vi "Mass Assign Window Text.vi"() -> ()   [LabVIEW 2023]
uses:
  9ee1baf5-252d-4dbe-adf5-4428d1966d26.vi
  96e9d38a-46f1-45bd-90ed-3046ef3e3c05.vi
  <userlib>/_OpenG.lib/file/file.llb/openg_file.lvlib
panel:
  out "file paths":path[](array[path])
  out "error out":errorcluster
  out "N":i32
  out "i":i32
  in  "error in (no error)":errorcluster
  in  "Decal Root":path
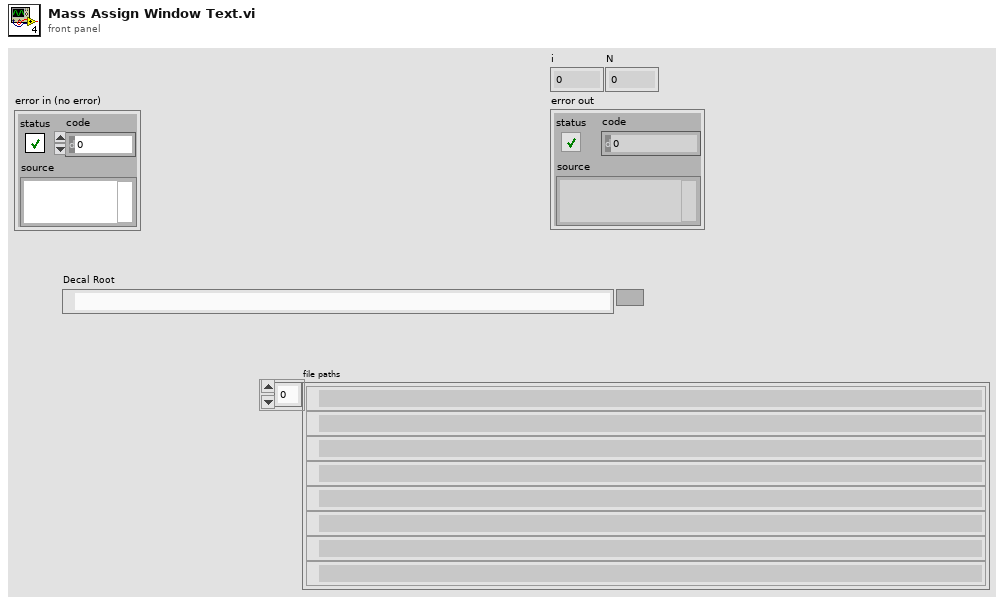
[diagram p1: front panel]
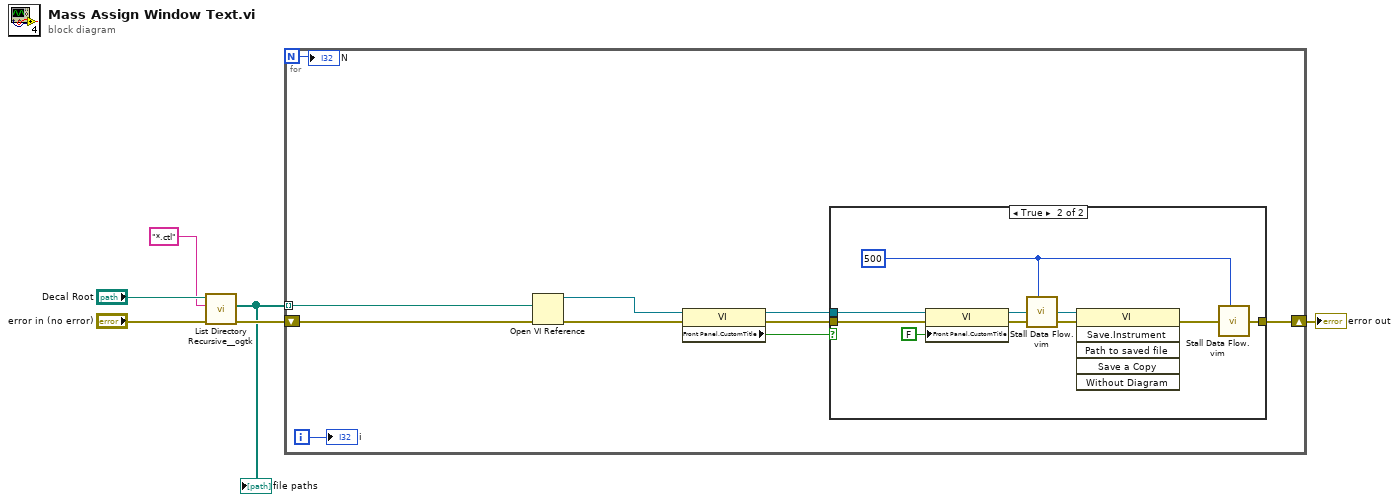
[diagram p0: block diagram]
diagram:
  n1 = call <userlib>:"List Directory Recursive__ogtk.vi"("error in (no error)"="error in (no error)", "pattern"="*.ctl", "Path"="Decal Root") -> ("error out"=w3:errorcluster, "file paths"=w2:path[])  [unwired: 5 in, 2 out]
  "file paths" <- w2
  n2 = for {
    N -> [w15]
    tunnel: w2 -> [w13] mode=indexing
    shift-right: [w12] -> w1
    shift-left: w3 -> [w14]
    i -> [w16]
    n3 = Open VI Reference(vi path=w13, error in (no error)=w14) -> (vi reference=w11:refnum<vi>, error out=w8:errorcluster)  [unwired: 4 in]
    n4 = property class="VI"(reference=w11, error in=w8) -> (reference out=w10:refnum<vi>, error out=w9:errorcluster, "Front Panel.CustomTitle"=w7:bool)
    n5 = case shown="True" w7 {
      tunnel: [w17 w21] -> w12
      tunnel: w10 -> [_ w19]
      tunnel: w9 -> [w17 w18]
      frame False {
      }
      frame True {
        w20 = 500
        n6 = property class="VI"(reference=w19, error in=w18, "Front Panel.CustomTitle"=FALSE ("Front Panel Window:Custom Title")) -> (reference out=w23:refnum<vi>, error out=w25:errorcluster)
        n7 = call "Stall Data Flow.vim"("value in"=w23, "milliseconds to wait"=w20) -> ("value out"=w22:refnum<vi>)  [unwired: 1 out]
        n8 = invoke class="VI" method="Save.Instrument"(reference=w22, error in=w25) -> (error out=w26:errorcluster)  [unwired: 4 in, 5 out]
        n9 = call "Stall Data Flow.vim"("value in"=w26, "milliseconds to wait"=w20) -> ("value out"=w21:errorcluster)  [unwired: 1 out]
      }
    }
    "i" <- w16
    "N" <- w15
  }
  "error out" <- w1
